vi "stage_idling_rapid.vi"(9 "num":u8, 10 "pos":dbl) -> ()   [LabVIEW 2019]
panel:
  out "string out":string
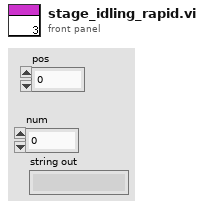
[diagram p1: front panel]
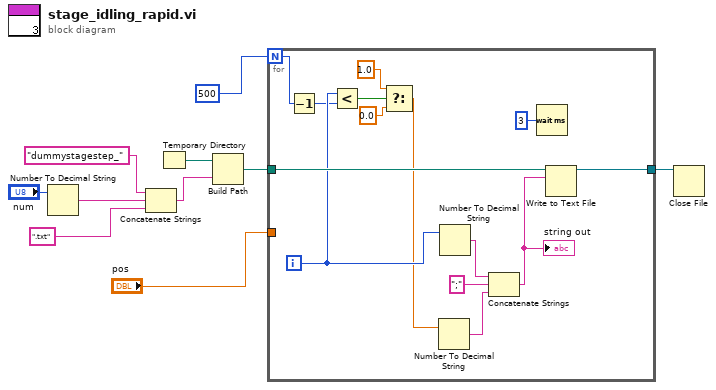
[diagram p0: block diagram]
diagram:
  n1 = Number To Decimal String(number="num") -> (decimal integer string=w6:string)  [unwired: 1 in]
  n2 = Concatenate Strings("dummystagestep_", w6, ".txt") -> (w4:string)
  n3 = Temporary Directory() -> (w2:path)
  n4 = Build Path(base path=w2, name or relative path=w4) -> (appended path=w3:path)
  n5 = for {
    N: 500 -> [w19]
    tunnel: "pos" -> [_]
    tunnel: [w24] -> w9
    tunnel: w3 -> [w23]
    i -> [w20]
    n6 = Decrement(x=w19) -> (x-1=w18:i32)
    n7 = Less?(x=w20, y=w18) -> (x < y?=w17:bool)
    n8 = Select(t=1.0, s=w17, f=0.0) -> (s? t:f=w14:dbl)
    n9 = Number To Decimal String(number=w14) -> (decimal integer string=w13:string)  [unwired: 1 in]
    n10 = Number To Decimal String(number=w20) -> (decimal integer string=w21:string)  [unwired: 1 in]
    n11 = Concatenate Strings(w21, ";", w13) -> (w12:string)
    "string out" <- w12
    n12 = Wait (ms)(milliseconds to wait=u32 3) -> ()  [unwired: 1 out]
    n13 = Write to Text File(file (use dialog)=w23, text=w12) -> (refnum out=w24:refnum<file>)  [unwired: 2 in, 2 out]
  }
  n14 = Close File(refnum=w9) -> ()  [unwired: 1 in, 2 out]
